vi "GaugeRampExample.vi"() -> ()   [LabVIEW 2010]
panel:
  in  "Blinking?":bool=TRUE
  out "Scale.Marker Values[] 2":cluster{dbl, u32}[](array[cluster])=[{0.0, 16711680}, {1.0, 6618880}, {2.0, 16711680}, {3.0, 0}] {"?" format="%#.6f"}
  in  "Scale.Marker Values[]":cluster{dbl, u32}[](array[cluster])=[{0.0, 16711680}, {1.0, 6618880}, {2.0, 16711680}, {3.0, 0}]
  in  "Supply Pressure":dbl(knob) scale=0.0..3.0
  # "Red = 16711680"
  # "Green = 6618880"
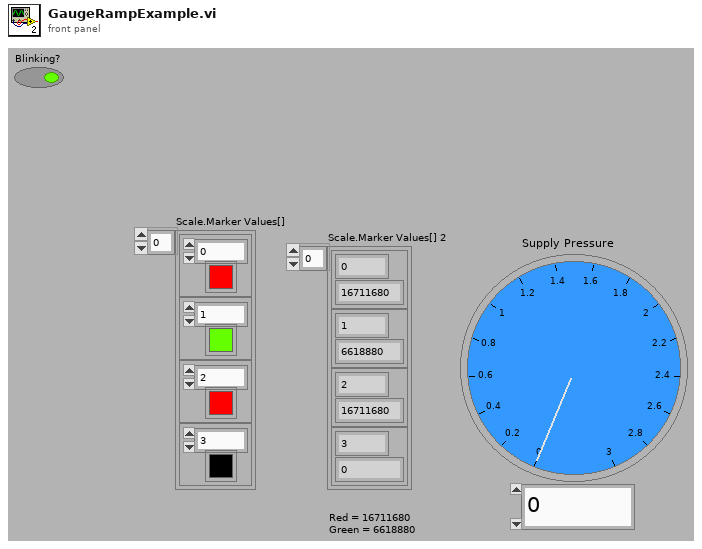
[diagram p1: front panel]
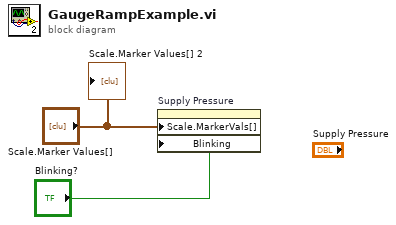
[diagram p0: block diagram]
diagram:
  n1 = property on="Supply Pressure" class="Knob (strict)"("Scale.MarkerVals[]"="Scale.Marker Values[]", "Blinking"="Blinking?") -> ()  [unwired: 2 in, 2 out]
  "Scale.Marker Values[] 2" <- "Scale.Marker Values[]"
